vi "peak - fit phase around center - V2.vi"(5 "Phase":dbl[](array[numeric]), 6 "VI Refnum":refnum<vi>, 7 "omega":dbl[](array[numeric]), 8 "weights":dbl[](array[numeric])=[0.0035625870091985437, 0.0035688503454743307, 0.0035799803322629988, 0.0035838407509538057, 0.0035856030846732785, 0.003587569380969158, 0.0035843086479959525, 0.0035835164661516938, 0.0035850008675947917, 0.0035837626329120837, 0.0035811679175952703, 0.0035784219376709748, 0.0035753719096975776, 0.0035727480013135436, 0.003571273109988151, 0.003565821664458903, 0.003562822105347891, 0.0035625604426215906, 0.00356229877989529, 0.0035620371171689895, 0.003561775454442689, 0.0035615137917163883, 0.0035612521289900877, 0.0035609904662637876, 0.0035607288035374874, 0.003560467140811187, 0.0035602054780848862, 0.0035599438153585856, 0.003559682152632285, 0.0035594204899059845, 0.003559158827179684, 0.0035588971644533837, 0.003558635501727083, 0.003558373839000783, 0.0035581121762744824, 0.003557850513548182, 0.0035575888508218812, 0.0035573271880955807, 0.00355706552536928, 0.00355680386264298, 0.0035565421999166793, 0.0035562805371903788, 0.0035560188744640786, 0.003555757211737778, 0.0035554955490114774, 0.003555233886285177, 0.0035549722235588763, 0.003554710560832576, 0.0035544488981062755, 0.003554187235379975, 0.003553925572653675, 0.003553663909927374, 0.0035534022472010736, 0.003553140584474773, 0.0035528789217484725, 0.003552617259022172, 0.0035523555962958717, 0.003552093933569571, 0.0035518322708432705, 0.0035515706081169704, 0.00355130894539067, 0.0035510472826643692, 0.0035507856199380686, 0.003550523957211768, 0.0035502622944854675, 0.0035500006317591673, 0.003549738969032867, 0.003549477306306566, 0.003549215643580266, 0.0035489539808539654, 0.003548692318127665, 0.0035484306554013642, 0.0035481689926750637, 0.0035479073299487635, 0.003547645667222463, 0.0035473840044961628, 0.003547122341769862, 0.0035468606790435616, 0.003546599016317261, 0.0035463373535909604, 0.00354607569086466, 0.0035458140281383593, 0.003545552365412059, 0.0035452907026857585, 0.0035450290399594584, 0.003544767377233158, 0.003544505714506857, 0.0035442440517805566, 0.003543982389054256, 0.003543720726327956, 0.003543459063601655, 0.0035431974008753547, 0.0035429357381490546, 0.003542674075422754, 0.0035424124126964534, 0.003542150749970153, 0.0035418890872438522, 0.0035416274245175516, 0.0035413657617912515, 0.003541104099064951, 0.0035408424363386503, 0.00354058077361235, 0.0035407248527083665, 0.0035406780052805913, 0.0035403792521782104, 0.003540557398401449, 0.0035402008071060216, 0.003539993309937548, 0.003540245806751373, 0.003540263900948342, 0.0035397789010768255, 0.003540037767688355, 0.0035397918231559753, 0.003539342760492389, 0.0035389265360938737, 0.003538492738838126, 0.003538621549531763, 0.003538118111061542, 0.0035380134349903046, 0.00353786420423612, 0.0035378829497169904, 0.0035376002922833825, 0.00353737374030193, 0.003537303240597115, 0.0035374213041562148, 0.00353706360898377, 0.003537396326021588, 0.003537133299738949, 0.00353683893508461, 0.0035368570675222413, 0.0035363147763650387, 0.0035364679965840346, 0.0035363445662985743, 0.0035371358675332673, 0.0035369739572430644, 0.0035365840463865757, 0.003536882856640864, 0.003536971396789569, 0.0035374492570215653, 0.003537644357907623, 0.0035374384190503642, 0.0035377406347297646, 0.003537653440536446, 0.003537756619944432, 0.0035374422299090007, 0.0035377498389208757, 0.0035380977090296445, 0.0035379188096958166, 0.0035380042137668965, 0.003538452671501436, 0.00353819038969424, 0.0035388271874688057, 0.0035394664694802618, 0.003539439059317983, 0.0035389722289594543, 0.0035392065121368577, 0.0035394439281405806, 0.003539235702593656, 0.003539978900751624, 0.003540024010459605, 0.003539811240342784, 0.0035398296079046923, 0.0035403679293004287, 0.0035410087522947417, 0.003541208704167959, 0.003541294869304514, 0.003542089137564577, 0.003542220731932116, 0.003542571193281065, 0.003543137689228242, 0.003543328114140262, 0.0035432335633283764, 0.0035431338106369156, 0.0035435204871514694, 0.0035437373108573606, 0.0035436341387524873, 0.0035436962919763344, 0.0035442557189842637, 0.0035441910740509454, 0.0035444539769206316, 0.003544218716671544, 0.003544643410492294, 0.003544678006805517, 0.0035454369747882674, 0.003545539290313343, 0.003545147340797882, 0.0035452602330044037, 0.0035454677574130035, 0.0035455949570138917, 0.003545939168811464, 0.003546114471589525, 0.0035462863898945603, 0.0035455927389847694, 0.0035454638860674156, 0.003545760573561209, 0.003545575904833474, 0.0035456174134914607, 0.0035454820849638, 0.003545573314678251, 0.0035456736703418914, 0.0035453882166531104, 0.0035457882443811293, 0.0035461608572059417, 0.0035460336858503896, 0.0035457041250836494, 0.003545779513003054, 0.0035454316197350826, 0.003545116544116847, 0.0035451781238433067, 0.0035449411657253968, 0.00354501505081026, 0.0035448580464249478, 0.003544198459951312, 0.0035440533677767285, 0.0035439917358835427, 0.00354351111774959, 0.0035434986894752277, 0.0035422738476958765, 0.003541588092290983, 0.0035410306041224163, 0.003540622950666575, 0.0035406596646636785, 0.00354046804819428, 0.003543722881933678, 0.0035540531654730976, 0.003572081265234354, 0.0035904401698712363, 0.0036079299287176793, 0.0036234759838145755, 0.003624761919214058, 0.003625792343897806, 0.003627365528749319, 0.0036285692231568327, 0.003630078850620531, 0.003615122915121112, 0.0036163976954264035, 0.003617729027545759, 0.0036181868899870617, 0.0036195096760864645, 0.003620920669601705, 0.003602217502409103, 0.003603099658199955, 0.0036041684052611263, 0.003604797382963272, 0.003605982935195567, 0.003607387128602013, 0.0036079456896162326, 0.003608917152439218, 0.0036104326626868926, 0.003611267220550441, 0.003588884169733501, 0.0035900360710838276, 0.0035907040603513187, 0.0035918592701429594, 0.0035936517771510057, 0.003594119326778623, 0.0035946261719768664, 0.0035958030184319936, 0.0035959713729800565, 0.003569557108412738, 0.0035695923946830123, 0.0035692285543541093, 0.003569182119424985, 0.0035700880490618977, 0.0035698258199099303, 0.0035704161529211886, 0.0035526869958115506, 0.003570965636529928, 0.0035523560164258125, 0.003572419450390771, 0.0035531879741292315, 0.003553691199040588, 0.003553540553052189, 0.0035532183547257574, 0.003552747738369849, 0.0035458936354283085, 0.0035520375754291185, 0.003545521872965046, 0.003552111864697351, 0.00354392954916202, 0.0035427999828177093, 0.0035411604354127066, 0.0035403962176682115, 0.0035403027417202342, 0.0035393465540448843, 0.003537961400212195, 0.0035367483951148433, 0.0035348097590437184, 0.0035332941609380573, 0.003531413945821079, 0.003528879058505537, 0.0035276852664089878, 0.0035247859776086545, 0.0035231317871338235, 0.003519006323367564, 0.0035172652295312845, 0.0035147959173586025, 0.00351255114841543, 0.0035108842389118865, 0.0035072639199511795, 0.003505758545454204, 0.0035010198565802847, 0.0034958190758545924, 0.003492878115765016, 0.003488238935994356, 0.0034826027627013973, 0.0034783159123673575, 0.0034769273689347, 0.0034724616998637195, 0.003467262239573098, 0.0034619621712673222, 0.0034574441596964896, 0.0034486864226109465, 0.003442459750297909, 0.0034387630861745086, 0.00344340035386684, 0.0034230698013945652, 0.0034366907267889078, 0.0034464767267684106, 0.0034496612873088665, 0.0034764400425292196, 0.003508312971236857, 0.004003505366835951, 0.005446448201245334, 0.007015224327135097, 0.0073193064503082675, 0.007020015415624015, 0.006636224018254199, 0.00635007764010221, 0.0061015396577520555, 0.005878799754674854, 0.005671783048105356, 0.005495510075695435, 0.005316033114439092, 0.005190239469835224, 0.005033415798309496, 0.004895500883285887, 0.00475610445184947, 0.004621137370117735, 0.004530918455433998, 0.004414139332582437, 0.004349021755846054, 0.004282057457066873, 0.004243058130876325, 0.004189349008410379, 0.004132829581662659, 0.004125887975536832, 0.004090541642406664, 0.004054303689620724, 0.00402291539948009, 0.004001095682415176, 0.00398685197445568, 0.003967716870320777, 0.003958412020907138, 0.00394063674640206, 0.003930916342756457, 0.003919856942414786, 0.0039045755802475293, 0.003889506766900452, 0.0038725481325029157, 0.0038569673361774828, 0.0038451756664663614, 0.003837285819041418, 0.0038311153095985577, 0.0038196279157010123, 0.0038154663513020977, 0.00380802490135134, 0.0037990162346051353, 0.0037909324976643363, 0.0037845104887504893, 0.0037818500807272303, 0.00377302640422651, 0.003767084133647707, 0.0037656781208253486, 0.003764410549630827, 0.003759908044084384, 0.00375710810133189, 0.00375351852657178, 0.0037496157613987205, 0.003749257205601429, 0.003749298681460832, 0.003747472623490328, 0.003745635382417998, 0.0037422456213832083, 0.003740110343124966, 0.0037384892224267083, 0.0037406774950601634, 0.003738787968320024, 0.0037372691914901645, 0.003734656298792755, 0.0037321712862071936, 0.0037297320968776217, 0.003730747884878853, 0.003728172516374503, 0.003725618663389812, 0.0037232013372860383, 0.0037206295999788457, 0.0037179433941660744, 0.003715689990982847, 0.003714059179831356, 0.003711467321429794, 0.003711940032664343, 0.0037103868584477963, 0.003707217638012632, 0.0037053165823798095, 0.0037031803081765844, 0.00370125762114856, 0.003698535390587881, 0.0036971229311498466, 0.0036983079614138622, 0.003695895306506089, 0.003693541990264217, 0.003690687001295564, 0.00368899626845673, 0.003687542625064116, 0.003685099734093935, 0.003683286051446689, 0.00368122605479984, 0.003679504884572229, 0.003677948740996124, 0.0036763650955602004, 0.0036741852680567243, 0.0036723219320306325, 0.0036709983766397445, 0.003669378697262484, 0.003667335711732546, 0.0036652856049053974, 0.0036634288409643527, 0.003661728855185431, 0.0036602842285372132, 0.003658847418809513, 0.0036568374589429128, 0.003655393158101771, 0.0036534509962713787, 0.0036515652247753935, 0.003649860145654834, 0.0036485601790056618, 0.003646585193220708, 0.0036452816783861678, 0.0036439748750041285, 0.0036420232657352935, 0.0036402336996620103, 0.0036391121453762873, 0.003637552072780926, 0.0036365946034344204, 0.003633338794896165, 0.0036305610563928834, 0.0036273704725145093, 0.003624589865660734, 0.0036217997787635356, 0.0036190095240981857, 0.0036170848561178667, 0.003614851850080103, 0.0036124063463852194, 0.0036107248894119946, 0.003608226217699194, 0.003606589434156585, 0.0036043090788185875, 0.003602588921929874, 0.003600951125959464, 0.003598596154086047, 0.003597422593005055, 0.003595448616291688, 0.003593651011148659, 0.003591956118153282, 0.0035904785246233927, 0.0035897505995611287, 0.003587670013565459, 0.003586121669890769, 0.0035851062161595185, 0.003583964586048097, 0.0035831329918504335, 0.003581710560383311, 0.003580981707491795, 0.003580442585718136, 0.0035786304566435513, 0.003578505180216165, 0.003577908489337322, 0.003576804437535286, 0.0035753353096396314, 0.0035740283471956836, 0.0035732576151722793, 0.0035720595315749584, 0.0035716298387044663, 0.0035711825490205296, 0.0035694130952146647, 0.003569068853640023, 0.003568341829649417, 0.003567861073326771, 0.003566883222673176, 0.0035654754232499856, 0.0035650819356715657, 0.003563700589137289, 0.003562945852908281, 0.0035620635471613395, 0.003561284266695623, 0.0035609326161442478, 0.0035593432184843547, 0.0035586750395117574, 0.0035576792989075517, 0.0035563663133494055, 0.003556031001436844, 0.003554949376725818, 0.003553916242438686, 0.00355300755342564, 0.0035520988644125928, 0.003551190175399546, 0.0035502814863864994, 0.0035493727973734523, 0.003548464108360406, 0.003547555419347359, 0.003546646730334312, 0.0035457380413212655, 0.0035448293523082184, 0.003543920663295172, 0.003543011974282125, 0.0035421032852690783, 0.0035411945962560316, 0.0035402859072429845, 0.0035393772182299383, 0.003538468529216891, 0.0035375598402038444, 0.0035366511511907978, 0.0035357424621777506, 0.0035348337731647044, 0.0035339250841516573, 0.0035330163951386106, 0.003532107706125564, 0.0035311990171125168, 0.00353029032809947, 0.0035293816390864234, 0.0035284729500733767, 0.00352756426106033, 0.003526655572047283, 0.003525746883034236, 0.0035248381940211895, 0.003523929505008143, 0.003523020815995096, 0.003522112126982049, 0.0035212034379690023, 0.0035202947489559556, 0.003519386059942909, 0.0035184773709298622, 0.003517568681916815, 0.0035166599929037684, 0.0035157513038907217, 0.003514842614877675, 0.0035139339258646284, 0.0035130252368515812, 0.0035121165478385345, 0.003511207858825488, 0.0035102991698124407, 0.0035093904807993945, 0.0035084817917863474, 0.0035075731027733007, 0.003506664413760254, 0.003505755724747207, 0.0035048470357341606, 0.0035039383467211135, 0.0035030296577080668, 0.00350212096869502, 0.003501212279681973, 0.0035003035906689267, 0.0034993949016558796, 0.003498486212642833, 0.003497577523629786, 0.003496668834616739, 0.003495760145603693, 0.0034948514565906457, 0.003493942767577599, 0.0034930340785645523, 0.003492125389551505, 0.003491216700538459, 0.003490308011525412, 0.003489399322512365, 0.0034884906334993184, 0.0034875819444862713, 0.003486673255473225, 0.003485764566460178, 0.003484855877447131, 0.0034839471884340846, 0.0034830384994210374, 0.0034821298104079908, 0.003481221121394944, 0.003480312432381897, 0.0034794037433688503, 0.0034784950543558036, 0.0034775863653427564, 0.00347667767632971, 0.003475768987316663, 0.0034748602983036164, 0.0034739516092905697, 0.0034730429202775226, 0.0034721342312644763, 0.003471225542251429, 0.0034703168532383825, 0.003469408164225336, 0.0034684994752122887, 0.0034675907861992424, 0.0034666820971861953, 0.0034657734081731486, 0.003464864719160102, 0.003463956030147055, 0.0034630473411340085, 0.005233304275841307], 9 "guess at theta":dbl, 10 "guess at gamma":dbl, 11 "guess at omega":dbl) -> (1 "fit for theta":dbl, 2 "fit for gamma":dbl, 3 "fit for omega":dbl)   [LabVIEW 2018]
uses:
  <vilib>/gmath/NI_Gmath.lvlib
  <vilib>/gmath/NumericalOptimization/Nonlinear Curve Fit LM.vi
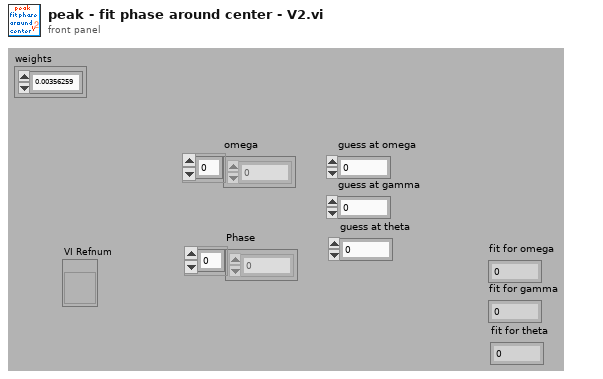
[diagram p1: front panel]
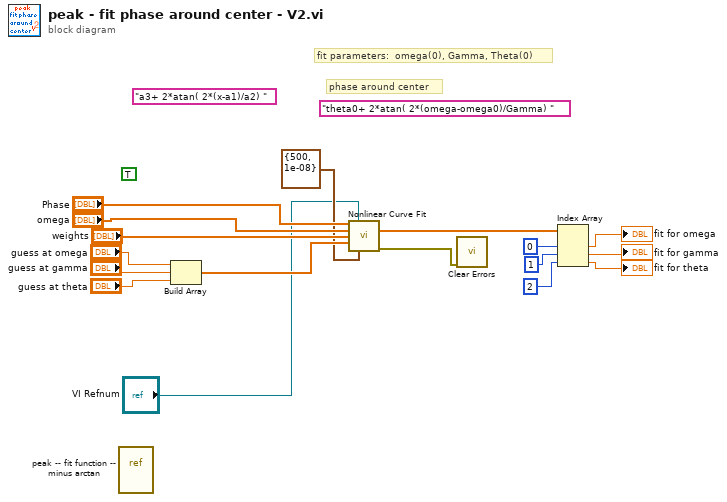
[diagram p0: block diagram]
diagram:
  (unwired) TRUE
  (unwired) "a3+ 2*atan( 2*(x-a1)/a2) " ("model")
  (unwired) "theta0+ 2*atan( 2*(omega-omega0)/Gamma) " ("model")
  # "fit parameters:  omega(0), Gamma, Theta(0)"
  # "phase around center"
  n1 = vi-ref "peak -- fit function -- minus arctan.vi"() -> ()  [unwired: 1 out]
  n2 = Build Array("guess at omega", "guess at gamma", "guess at theta") -> (w8:dbl[])
  n3 = call-poly <vilib>:"Nonlinear Curve Fit.vi"("Y"="Phase", "f(x,a)"="VI Refnum", "X"="omega", "Weight"="weights", "initial parameters"=w8, "termination"=cluster{"max iteration":i32, "tolerance":dbl} {"max iteration"=500, "tolerance"=1e-08}) -> ("best fit parameters"=w7:dbl[], "error out"=w3:errorcluster)  [unwired: 4 in, 4 out]
  n4 = call <vilib>:"Clear Errors.vi"("error in (no error)"=w3) -> ()  [unwired: 5 in, 2 out]
  n5 = Index Array(array=w7, index #1=0, index #2=1, index #3=2) -> (element #1=→"fit for omega":dbl, element #2=→"fit for gamma":dbl, element #3=→"fit for theta":dbl)
